vi "PDFL1dll.vi"(8 "error in (no error)":errorcluster, 11 "Inputs":cluster{"p":dbl, "d":dbl, "z":dbl[], "t":dbl}) -> (0 "error out":errorcluster, 3 "Outputs":T1)   [LabVIEW 2021]
doc: "void __cdecl PDFL1dll(double *p, double *d, double *x, double *t, long *ierr, char herr[255], long ln);"
uses:
  REFPROP.dll
panel:
  # "REFPROP-PDFL1dll.vi"
  # "void  PDFL1dll(double *p, double *d, double *z, double *t, int32_t *ierr, CStr herr, int32_t herr_length);"
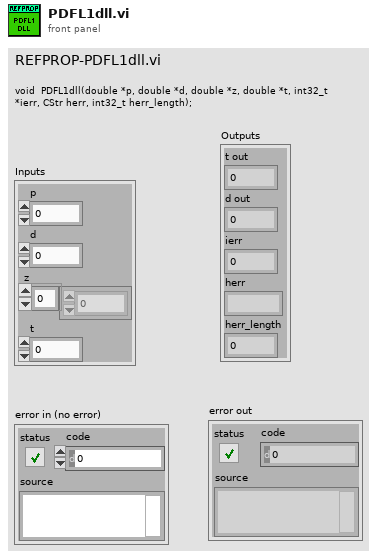
[diagram p1: front panel]
types:
  T1 = cluster{"t out":dbl, "d out":dbl, "ierr":i32, "herr":string, "herr_length":i32}
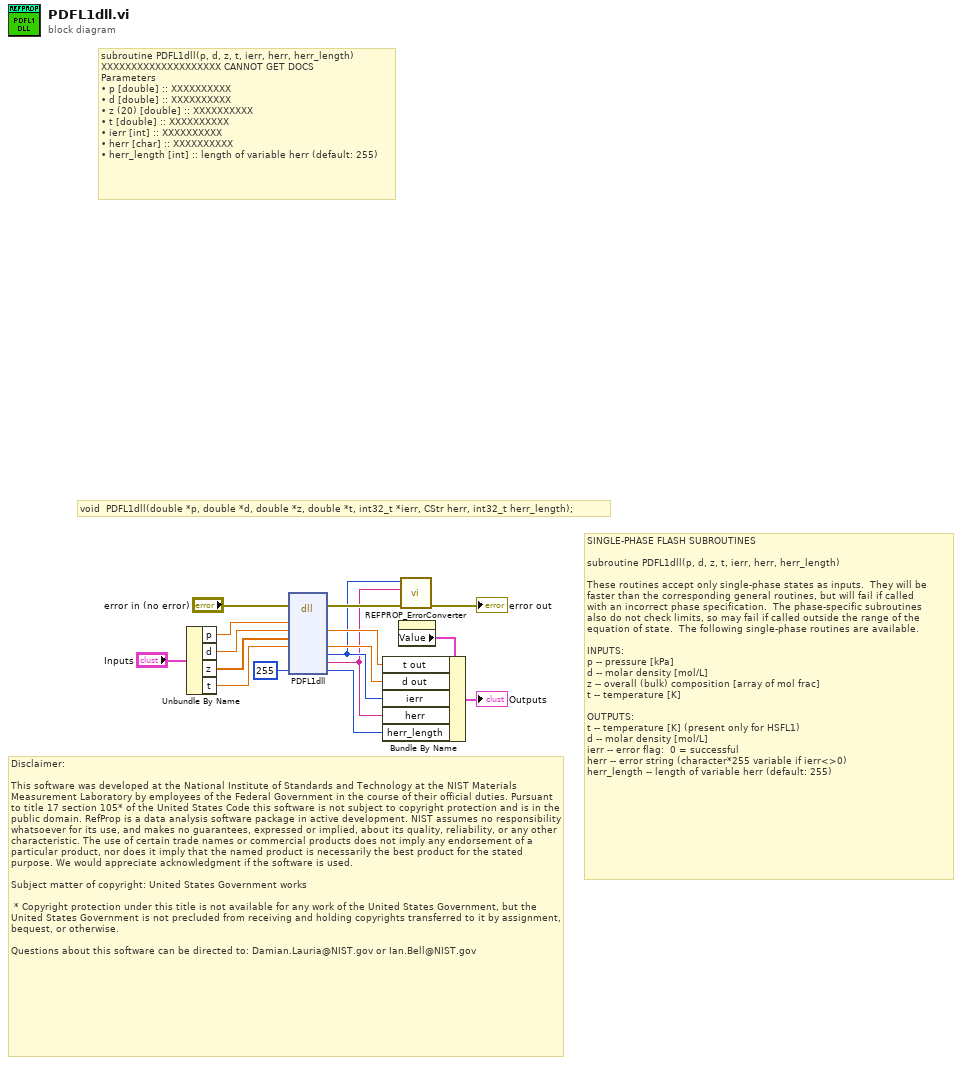
[diagram p0: block diagram]
diagram:
  # "Disclaimer:\n\nThis software was developed at the National Institute of Standards and Technology at the NIST Materials Measurement Laboratory by employees of the Federal Government in the course of their official duties. Pursuant to title 17 section 105* of the United States Code this software is not subject to copyright protection and is in the public domain. RefProp is a data analysis software package in active development. NIST assumes no responsibility whatsoever for its use, and makes no guarantees, expressed or implied, about its quality, reliability, or any other characteristic. The use of certain trade names or commercial products does not imply any endorsement of a particular product, nor does it imply that the named product is necessarily the best product for the stated purpose. We would appreciate acknowledgment if the software is used.\n \nSubject matter of copyright: United States Government works\n  \n * Copyright protection under this title is not available for any work of the United States Government, but the United States Government is not precluded from receiving and holding copyrights transferred to it by assignment, bequest, or otherwise.\n\nQuestions about this software can be directed to: Damian.Lauria@NIST.gov or Ian.Bell@NIST.gov"
  # "void  PDFL1dll(double *p, double *d, double *z, double *t, int32_t *ierr, CStr herr, int32_t herr_length);"
  # "subroutine PDFL1dll(p, d, z, t, ierr, herr, herr_length)\nXXXXXXXXXXXXXXXXXXXX CANNOT GET DOCS\nParameters\n• p [double] :: XXXXXXXXXX\n• d [double] :: XXXXXXXXXX\n• z (20) [double] :: XXXXXXXXXX\n• t [double] :: XXXXXXXXXX\n• ierr [int] :: XXXXXXXXXX\n• herr [char] :: XXXXXXXXXX\n• herr_length [int] :: length of variable herr (default: 255)"
  # "SINGLE-PHASE FLASH SUBROUTINES\n\nsubroutine PDFL1dll(p, d, z, t, ierr, herr, herr_length)\n\nThese routines accept only single-phase states as inputs.  They will be\nfaster than the corresponding general routines, but will fail if called\nwith an incorrect phase specification.  The phase-specific subroutines\nalso do not check limits, so may fail if called outside the range of the\nequation of state.  The following single-phase routines are available.\n\nINPUTS: \np -- pressure [kPa]\nd -- molar density [mol/L]\nz -- overall (bulk) composition [array of mol frac]\nt -- temperature [K]\n\nOUTPUTS:\nt -- temperature [K] (present only for HSFL1)\nd -- molar density [mol/L]\nierr -- error flag:  0 = successful\nherr -- error string (character*255 variable if ierr<>0)\nherr_length -- length of variable herr (default: 255)"
  n1 = Unbundle By Name("Inputs") -> ("p"=w10:dbl, "d"=w9:dbl, "z"=w8:dbl[], "t"=w7:dbl)
  n2 = dll-call lib="C:/Users/lauria/OneDrive - National Institute of Standards and Technology (NIST)/LabVIEW Projects/7 REFPROP/REFPROP-wrappers-master/REFPROP-wrappers-master/wrappers/Labview/REFPROP/REFPROP.*" fn="PDFL1dll"(error in="error in (no error)", "p"=w10, "d"=w9, "z"=w8, "t"=w7, "herr_length"=255) -> (error out=w16:errorcluster, "d"=w5:dbl, "t"=w4:dbl, "ierr"=w3:i32, "herr"=w2:string, "herr_length"=w1:i32)  [unwired: 7 in, 1 out]
  n3 = property on="Outputs" class="Clust (strict)"() -> ("Value"=w6:T1)  [unwired: 2 in, 2 out]
  n4 = Bundle By Name(cluster=w6, "t out"=w5, "d out"=w4, "ierr"=w3, "herr"=w2, "herr_length"=w1) -> (→"Outputs":T1)
  n5 = call "REFPROP_ErrorConverter.vi"("error in (no error)"=w16, "Error Message"=w2, "Error Code"=w3) -> ("error out"=→"error out":errorcluster)  [unwired: 8 in]
